vi "Set AO Data Value (automation mode).vi"(8 "error in (no error)":errorcluster, 9 "Value":dbl, 10 "AO IOName":string, 11 "DAQ":refnum<class "DAQ.lvclass">) -> (0 "error out":errorcluster, 3 "DAQ":refnum<class "DAQ.lvclass">)   [LabVIEW 2017, in "DAQ.lvclass"]
doc: "Developed by Kevin Thompson\nkevin@thompsonengineering.net\n\nCopyright 2018-2020\nThompson Engineering, LLC\nCall this Set AO Data Value method for setting analog output values in test modules that are executed during automatic testing."
uses:
  DAQ.lvclass
  DataTypes/TD DAQ Output EventSenderMode-enum.ctl
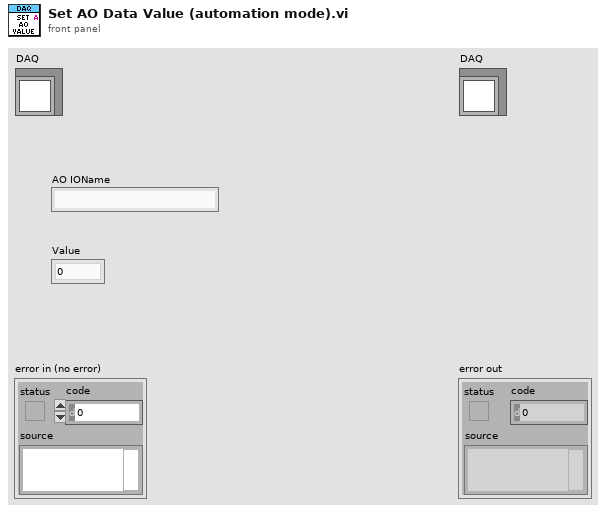
[diagram p1: front panel]
types:
  T1 = typedef "DAQ.lvclass/TD DAQ Output EventSenderMode-enum.ctl" = enum16{"manual", "automation"}
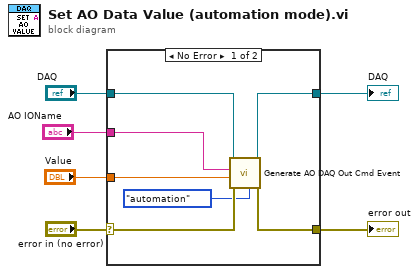
[diagram p0: block diagram]
diagram:
  n1 = case shown="No Error" "error in (no error)" {
    selector: "error in (no error)" -> [w13 w15]
    tunnel: [w12 w15] -> w5
    tunnel: [w10 w14] -> w3
    tunnel: "DAQ" -> [w11 w14]
    tunnel: "AO IOName" -> [w8 _]
    tunnel: "Value" -> [w7 _]
    frame No Error {
      n2 = call "Generate AO DAQ Out Cmd Event.vi"("mode (manual)"=TD_DAQ_Output_EventSenderMode-enum."automation", "error in (no error)"=w13, "AnalogVal"=w7, "AO IOName"=w8, "DAQ"=w11) -> ("error out"=w12:errorcluster, "DAQ"=w10:refnum<class "DAQ.lvclass">)  [unwired: 5 in]
    }
    frame Error {
    }
  }
  "error out" <- w5
  "DAQ" <- w3
